vi "channeldata_2ch_floatbigendianinterleaved.vi"() -> ()   [LabVIEW 2019]
panel:
  out "Error Out":errorcluster
  in  "TDMS File":path=path "C:/Python/projects/nitdms/tests/tdms_files/channeldata_2ch_floatbigendianinterleaved.tdms"
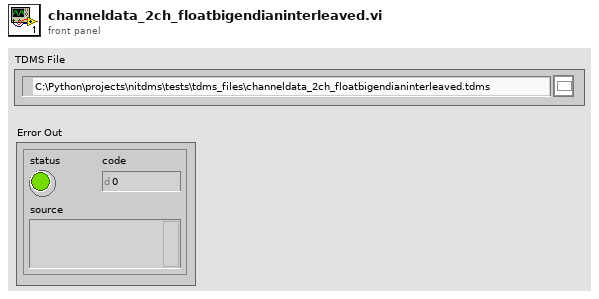
[diagram p1: front panel]
types:
  T1 = enum16{"big-endian, network order", "native, host order", "little-endian"}
  T2 = enum16{"open", "open or create", "create or replace", "create", "open (read-only)"}
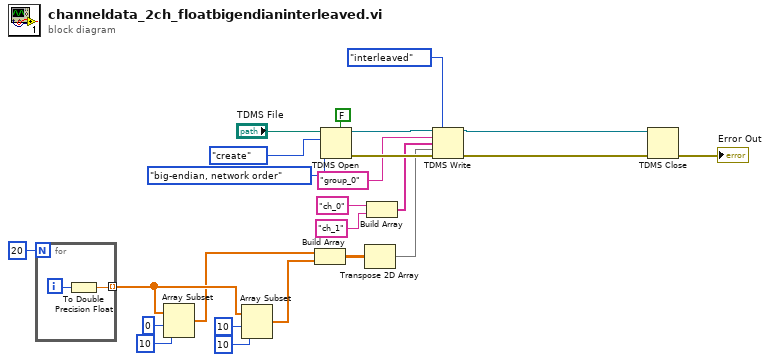
[diagram p0: block diagram]
diagram:
  n1 = for {
    N: 20 -> [_]
    tunnel: [w25] -> w12 mode=indexing
    i -> [w26]
    n2 = To Double Precision Float(number=w26) -> (double precision float=w25:dbl)
  }
  n3 = Array Subset(array=w12, index=0, length=10) -> (w11:dbl[])
  n4 = Array Subset(array=w12, index=10, length=10) -> (w10:dbl[])
  n5 = Build Array(w11, w10) -> (w3:dbl[][])
  n6 = TDMS Open(5:FALSE ("create index file? (T)"), 9:T1."big-endian, network order" ("byte order (2:little-endian)"), 10:T2."create" ("operation (0:open)"), 11:"TDMS File") -> (0:w20:errorcluster, 3:w19:refnum<k34>)  [unwired: 3 in]
  n7 = Transpose 2D Array(2D array=w3) -> (transposed array=w2:dbl[][])
  n8 = Build Array("ch_0", "ch_1") -> (w7:string[])
  n9 = TDMS Write(0:w19, 1:enum16{"decimated", "interleaved"}."interleaved" ("data layout (0:decimated)"), 5:"group_0", 7:w7, 9:w2, 11:w20) -> (4:w5:refnum<k34>, 15:w6:errorcluster)  [unwired: 2 out]
  n10 = TDMS Close(8:w6, 11:w5) -> (0:→"Error Out":errorcluster)  [unwired: 1 out]
